vi "AerotechStop.vi"(8 "error in (no error)":errorcluster) -> (0 "error out":errorcluster)   [LabVIEW 2009]
uses:
  Controls/AerotechCommand.ctl
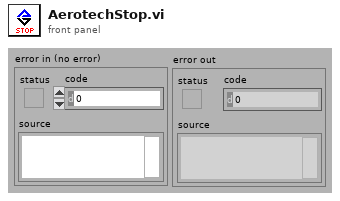
[diagram p1: front panel]
types:
  T1 = typedef "AerotechCommand.ctl" = enum16{"TRACK", "POSITION", "STOP", "HOME", "QUIT"}
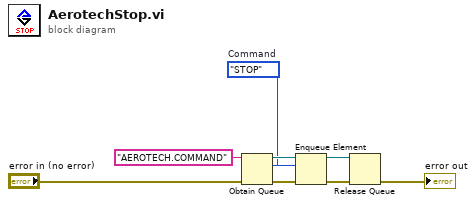
[diagram p0: block diagram]
diagram:
  w5 = AerotechCommand."STOP"  # Command
  n1 = Obtain Queue(name (unnamed)="AEROTECH.COMMAND", element data type=w5, error in (no error)="error in (no error)") -> (queue out=w6:refnum<queue>, error out=w7:errorcluster)  [unwired: 2 in, 1 out]
  n2 = Enqueue Element(queue=w6, element=w5, error in (no error)=w7) -> (queue out=w3:refnum<queue>, error out=w4:errorcluster)  [unwired: 1 in, 1 out]
  n3 = Release Queue(queue=w3, error in (no error)=w4) -> (error out=→"error out":errorcluster)  [unwired: 1 in, 2 out]
